vi "Get Address.vi"(8 "Error in":errorcluster, 11 "Address in":refnum<class "Address.lvclass">) -> (0 "Error out":errorcluster, 3 "Address out":refnum<class "Address.lvclass">)   [LabVIEW 2020, in "Address.lvclass"]
uses:
  Address.lvclass
  Address.lvclass/Address.ctl
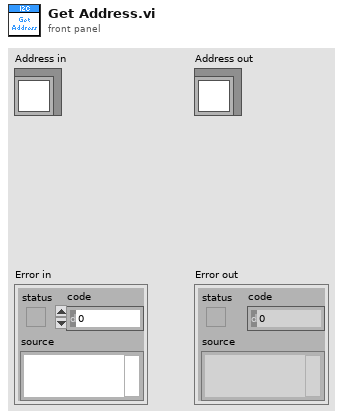
[diagram p1: front panel]
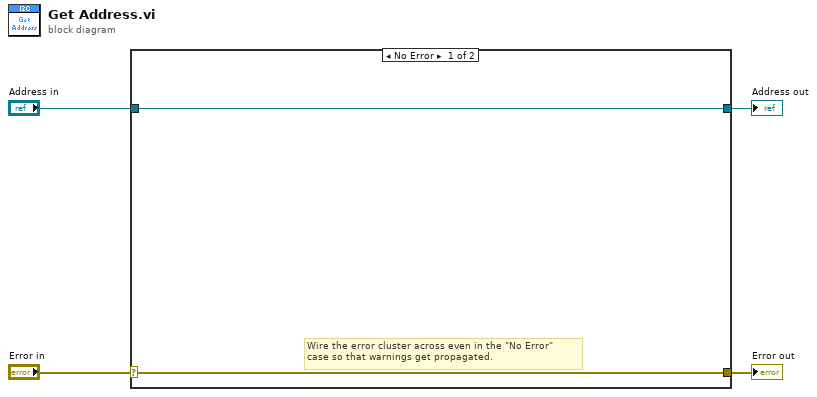
[diagram p0: block diagram]
diagram:
  n1 = case shown="No Error" "Error in" {
    selector: "Error in" -> [w5 w8]
    tunnel: [w5 w8] -> w3
    tunnel: [w6 w7] -> w1
    tunnel: "Address in" -> [w6 w7]
    frame No Error {
      # "Wire the error cluster across even in the \"No Error\"\ncase so that warnings get propagated."
    }
    frame Error {
    }
  }
  "Error out" <- w3
  "Address out" <- w1
